vi "Save Load Data.vi"(0 "[A/D Input]":dbl[][](array[numeric]), 5 "Shim #":i32, 7 "Eng-Result #":u32, 11 "error in (no error)":errorcluster, 12 "Re Create New Engr Results? (F)":bool, 13 "[Avg A/D Input]":dbl[][](array[numeric])) -> (4 "Pass?":bool, 6 "Error Code":i32, 8 "ScaleA":i32, 10 "ScaleB":i32, 15 "error out":errorcluster)   [LabVIEW 2015]
uses:
  <vilib>/addons/_office/excel.llb/Excel Easy Table (num).vi
  <vilib>/addons/_office/excel.llb/Excel Get Data (str).vi
  <vilib>/Utility/NIReport.llb/NI_report.lvclass
  <vilib>/addons/_office/NI_ReportGenerationToolkit.lvlib
  <vilib>/Utility/NIReport.llb/Excel/NI_Excel.lvclass
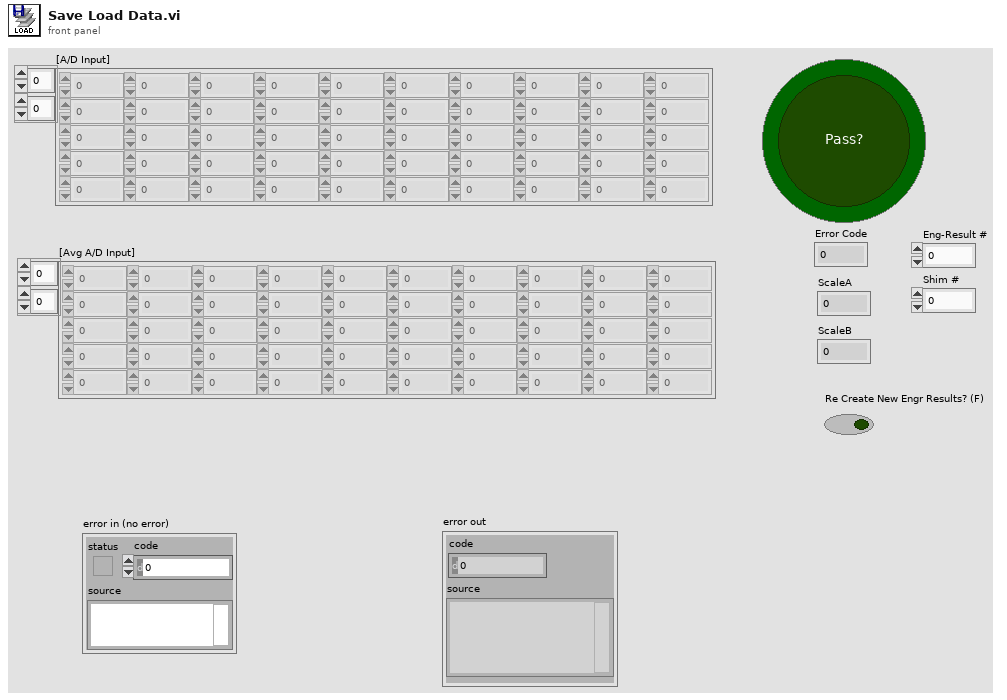
[diagram p1: front panel]
types:
  T1 = enum16{"maximized", "minimized", "normal", "no change"}
  T2 = enum16{"Standard Report", "HTML", "Word", "Excel"}
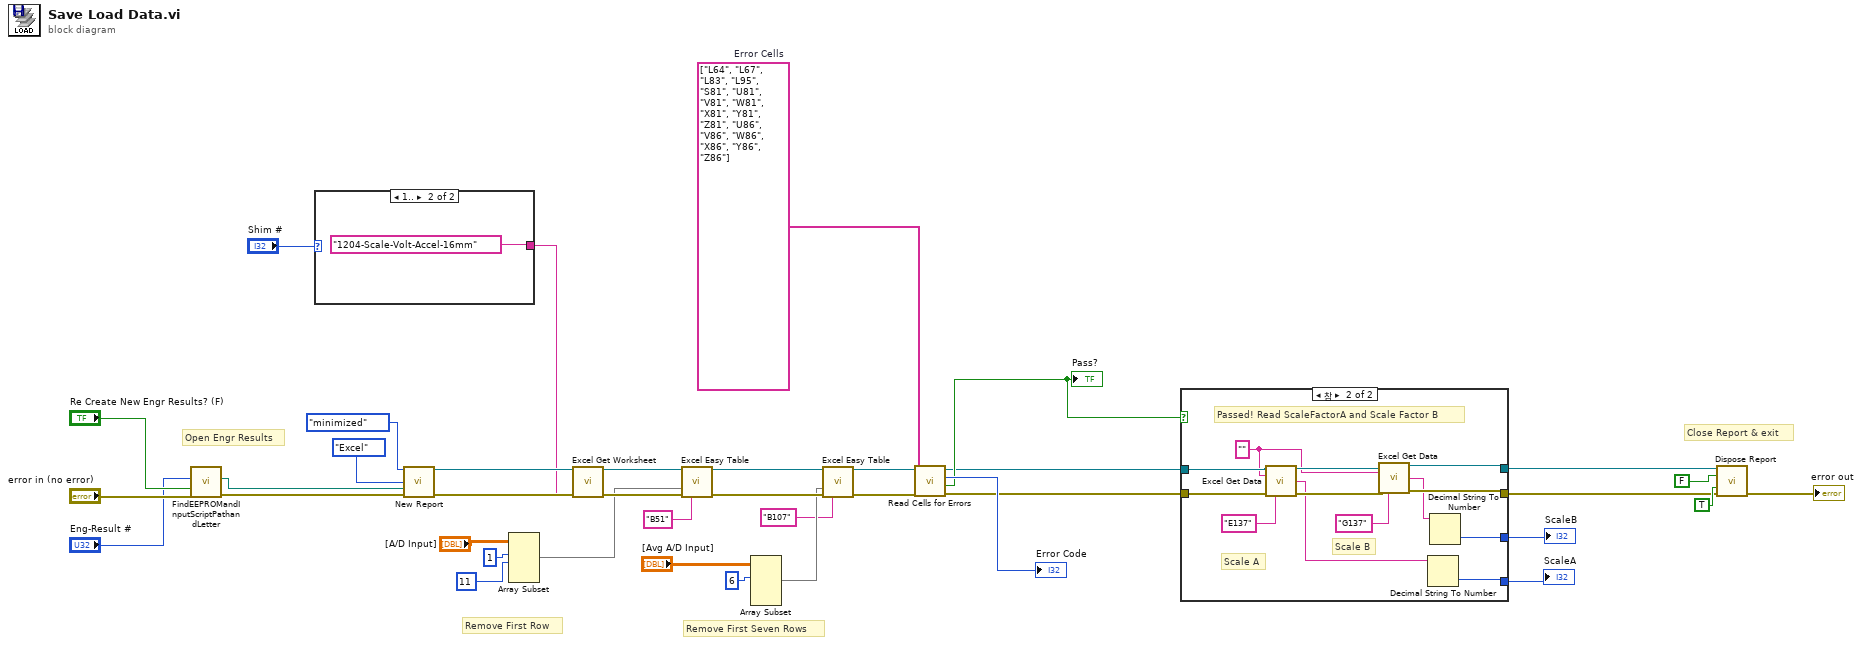
[diagram p0: block diagram]
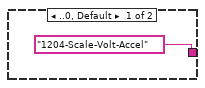
[diagram p2: hidden frame]
diagram:
  w23 = string[] ["L64", "L67", "L83", "L95", "S81", "U81", "V81", "W81", "X81", "Y81", "Z81", "U86", "V86", "W86", "X86", "Y86", "Z86"]  # Error Cells
  # "Remove First Seven Rows"
  # "Remove First Row"
  # "Close Report & exit"
  # "Open Engr Results"
  n1 = call "FindEEPROMandInputScriptPathandLetter.vi"("Error In"="error in (no error)", "Re Create New Engr Results? (F)"="Re Create New Engr Results? (F)", "Eng-Result #"="Eng-Result #") -> ("Error Out"=w29:errorcluster, "Engr Result Path"=w38:path)  [unwired: 4 in, 1 out]
  n2 = case shown="1.." "Shim #" {
    tunnel: ["1204-Scale-Volt-Accel" ("name (\"\")") "1204-Scale-Volt-Accel-16mm" ("name (\"\")")] -> w2
    frame ..0, Default {
    }
    frame 1.. {
    }
  }
  n3 = call <vilib>:"New Report.vi"("window state (normal)"=T1."minimized", "report type"=T2."Excel", "template (empty)"=w38, "error in (no error)"=w29) -> ("report out"=w32:refnum<class "NI_report.lvclass">, "error out"=w31:errorcluster)  [unwired: 10 in]
  n4 = Array Subset(array="[A/D Input]", index (row)=1 ("length"), length (row)=11 ("length")) -> (w22:dbl[][])  [unwired: 2 in]
  n5 = call <vilib>:"Excel Get Worksheet.vi"("report in"=w32, "error in (no error)"=w31, "name (\"\")"=w2) -> ("report out"=w28:refnum<class "NI_report.lvclass">, "error out"=w27:errorcluster)  [unwired: 11 in]
  n6 = call-poly <vilib>:"Excel Easy Table.vi"("report in"=w28, "text data"=w22, "error in (no error)"=w27, "name (\"\")"="B51" ("name (\"\")")) -> ("report out"=w11:refnum<class "NI_report.lvclass">, "error out"=w9:errorcluster)  [unwired: 7 in, 3 out]
  n7 = Array Subset(array="[Avg A/D Input]", index (row)=6 ("length")) -> (w5:dbl[][])  [unwired: 3 in]
  n8 = call-poly <vilib>:"Excel Easy Table.vi"("report in"=w11, "text data"=w5, "error in (no error)"=w9, "name (\"\")"="B107" ("name (\"\")")) -> ("report out"=w10:refnum<class "NI_report.lvclass">, "error out"=w8:errorcluster)  [unwired: 7 in, 3 out]
  n9 = call "Read Cells for Errors.vi"("error in (no error)"=w8, "Error Cells (ex:A12)"=w23, "NI_report in"=w10) -> ("error out"=w20:errorcluster, "Pass?"=w21:bool, "Error Code"=→"Error Code":i32, "NI_report out"=w19:refnum<class "NI_report.lvclass">)  [unwired: 5 in]
  "Pass?" <- w21
  n10 = case shown="참" w21 {
    tunnel: w20 -> [w41 w55]
    tunnel: w19 -> [w42 w54]
    tunnel: [w42 w51] -> w18
    tunnel: [w41 w50] -> w17
    tunnel: [_ w43] -> w16
    tunnel: [_ w44] -> w15
    frame False {
      # "Fail. No need to read the Scale Values"
    }
    frame True {
      w48 = "" ("name (\"\")")
      # "Scale A"
      # "Scale B"
      # "Passed! Read ScaleFactorA and Scale Factor B"
      n11 = call-poly <vilib>:"Excel Get Data.vi"("report in"=w54, "data type"=w48, "error in (no error)"=w55, "name (\"\")"="E137" ("name (\"\")")) -> ("report out"=w52:refnum<class "NI_report.lvclass">, "data"=w46:string, "error out"=w53:errorcluster)  [unwired: 9 in]
      n12 = call-poly <vilib>:"Excel Get Data.vi"("report in"=w52, "data type"=w48, "error in (no error)"=w53, "name (\"\")"="G137" ("name (\"\")")) -> ("report out"=w51:refnum<class "NI_report.lvclass">, "data"=w47:string, "error out"=w50:errorcluster)  [unwired: 9 in]
      n13 = Decimal String To Number(string=w46) -> (number=w43:i32)  [unwired: 2 in, 1 out]
      n14 = Decimal String To Number(string=w47) -> (number=w44:i32)  [unwired: 2 in, 1 out]
    }
  }
  "ScaleA" <- w16
  "ScaleB" <- w15
  n15 = call-dynamic "Dispose Report.vi"("report in"=w18, "wait until printing completed? (T)"=FALSE, "save changes? (F)"=TRUE, "error in (no error)"=w17) -> ("error out"=→"error out":errorcluster)  [unwired: 11 in]
